vi "DelayGeneratorGUI.vi"() -> ()   [LabVIEW 2009, in "DelayGenerator.lvlib"]
uses:
  DelayGenerator.lvlib
  Controls/Baseline.ctl
  Controls/SiteInformation.ctl
  Controls/StarAstrometricEntry.ctl
  Controls/DelayGeneratorState.ctl
panel:
  out "Offset":dbl[unit] format="%.6g"
  out "State":T1
  in  "IDLE Button":bool
  in  "TRACK Button":bool
  in  "Star Astrometric Entry":T2={"catalog"="HIP", "starname"="ANTARES", "starnumber"=80763, "ra"=59364.46079999999, "dec"=-0.4613254627937262, "promora"=-1.5608487288736407e-15, "promodec"=-3.565679035153268e-15, "parallax"=8.144869842640205e-09, "radialvelocity"=0.0} {"dec" format="%.6g"; "ra" format="%.6g"}
  in  "Location":T3={"latitude"=0.34599908001030344, "longitude"=-2.713521559899555, "height"=4123.0, "temperature"=0.0, "pressure"=0.0} {"longitude" format="%_10g"; "latitude" format="%_10g"}
  in  "Baseline":T4={"East"=0.0, "North"=2.0, "Up"=0.0} {"Up" format="%.6g"; "North" format="%.6g"; "East" format="%.6g"}
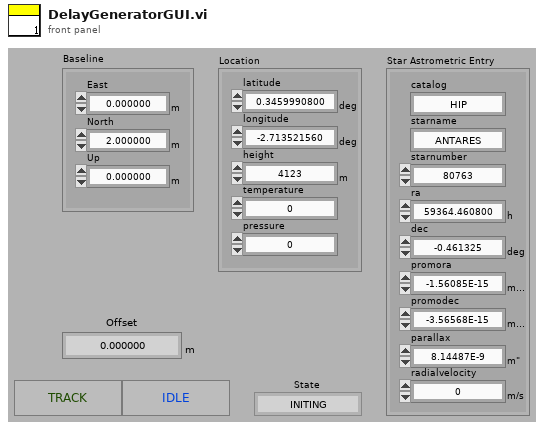
[diagram p1: front panel]
types:
  T1 = typedef "DelayGeneratorState.ctl" = enum16{"INITING", "IDLING", "TRACKING", "STOPPING"}
  T2 = typedef "StarAstrometricEntry.ctl" = cluster{"catalog":string, "starname":string, "starnumber":i32, "ra":dbl[unit], "dec":dbl[unit], "promora":dbl[unit], "promodec":dbl[unit], "parallax":dbl[unit], "radialvelocity":dbl[unit]}
  T3 = typedef "SiteInformation.ctl" = cluster{"latitude":dbl[unit], "longitude":dbl[unit], "height":dbl[unit], "temperature":dbl, "pressure":dbl}
  T4 = typedef "Baseline.ctl" = cluster{"East":dbl[unit], "North":dbl[unit], "Up":dbl[unit]}
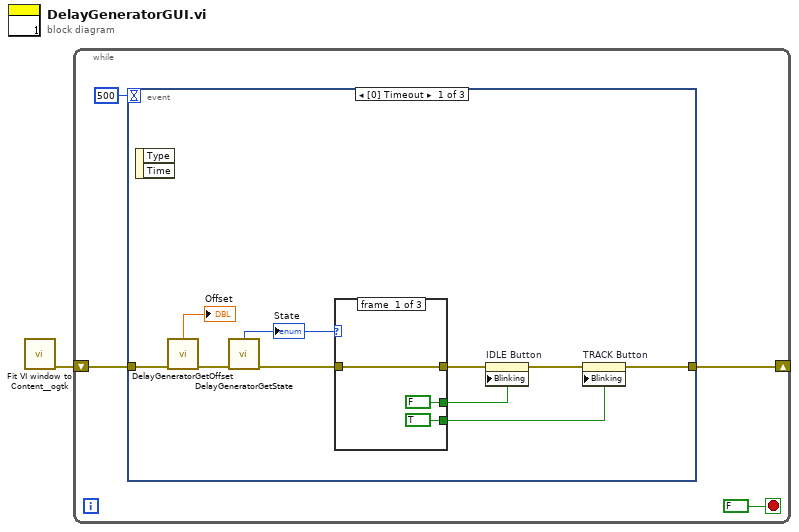
[diagram p0: block diagram]
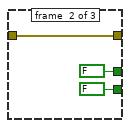
[diagram p2: hidden frame]
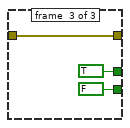
[diagram p3: hidden frame]
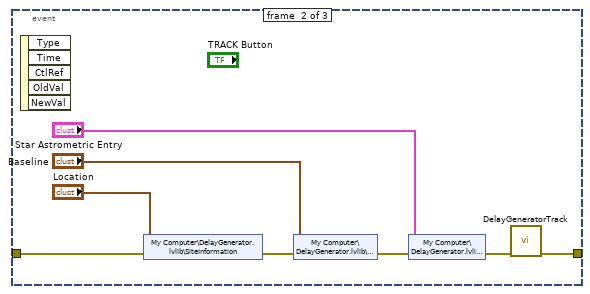
[diagram p4: hidden frame]
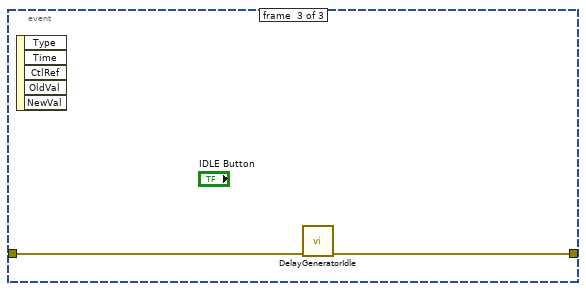
[diagram p5: hidden frame]
diagram:
  n1 = call <userlib>:"Fit VI window to Content__ogtk.vi"() -> ("error out"=w1:errorcluster)  [unwired: 6 in, 1 out]
  n2 = while {
    shift-right: [w5] -> _
    shift-left: w1 -> [w4]
    stop <- FALSE stop-if-true
    n3 = event shown="[0] Timeout" {
      selector: _ -> [_ _ _]
      dyn-events: _ -> [_ _ _]
      timeout: 500 -> [_ _ _]
      tunnel: w4 -> [w8 w27 w34]
      tunnel: [w14 w25 w33] -> w5
      event #0 {
        n4 = event-data() -> ()  [unwired: 1 in, 2 out]
        n5 = call "DelayGeneratorGetOffset.vi"("error in (no error)"=w8) -> ("Offset"=→"Offset":dbl[unit], "error out"=w7:errorcluster)  [unwired: 7 in]
        n6 = call "DelayGeneratorGetState.vi"("error in (no error)"=w7) -> ("State"=w12:T1, "error out"=w13:errorcluster)  [unwired: 7 in]
        "State" <- w12
        n7 = case shown="Default" w12 {
          tunnel: w13 -> [w18 w21 w24]
          tunnel: [w18 w21 w24] -> w11
          tunnel: [FALSE FALSE TRUE] -> w10
          tunnel: [TRUE FALSE FALSE] -> w9
          frame #0 {
          }
          frame #1 {
          }
          frame #2 {
          }
        }
        n8 = property on="IDLE Button" class="Bool"(error in=w11, "Blinking"=w10) -> (error out=w15:errorcluster)  [unwired: 1 in, 1 out]
        n9 = property on="TRACK Button" class="Bool"(error in=w15, "Blinking"=w9) -> (error out=w14:errorcluster)  [unwired: 1 in, 1 out]
      }
      event #1 {
        n10 = event-data() -> ()  [unwired: 1 in, 5 out]
        n11 = shared-variable "My Computer\\DelayGenerator.lvlib\\SiteInformation"("Location", error in=w27) -> (error out=w31:errorcluster)
        n12 = shared-variable "My Computer\\DelayGenerator.lvlib\\Baseline"("Baseline", error in=w31) -> (error out=w29:errorcluster)
        n13 = shared-variable "My Computer\\DelayGenerator.lvlib\\Target"("Star Astrometric Entry", error in=w29) -> (error out=w26:errorcluster)
        n14 = call "DelayGeneratorTrack.vi"("error in (no error)"=w26) -> ("error out"=w25:errorcluster)  [unwired: 10 in]
      }
      event #2 {
        n15 = event-data() -> ()  [unwired: 1 in, 5 out]
        n16 = call "DelayGeneratorIdle.vi"("error in (no error)"=w34) -> ("error out"=w33:errorcluster)  [unwired: 10 in]
      }
    }
  }
